vi "Set LabVIEW Server ID.vi"(7 "Server Alias":string, 10 "Error In":errorcluster, 11 "LabVIEW Server ID":string) -> (2 "Error Out":errorcluster)   [LabVIEW 2013, in "TS.lvlib"]
uses:
  TS.lvlib
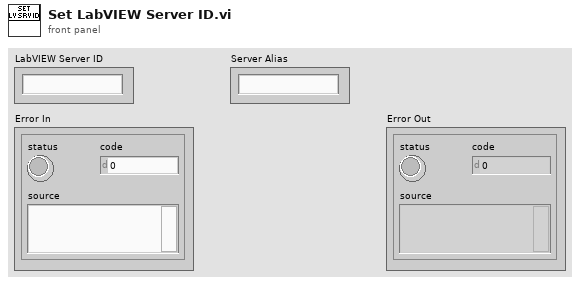
[diagram p1: front panel]
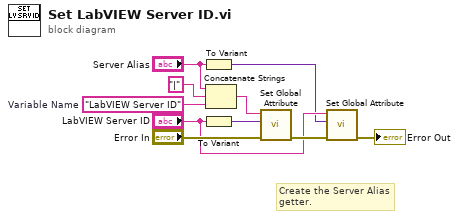
[diagram p0: block diagram]
diagram:
  w8 = "LabVIEW Server ID"  # Variable Name
  # "Create the Server Alias\ngetter."
  n1 = To Variant(anything="Server Alias") -> (Variant=w2:variant)
  n2 = To Variant(anything="LabVIEW Server ID") -> (Variant=w6:variant)
  n3 = Concatenate Strings("Server Alias", "|" ("string"), w8) -> (w7:string)
  n4 = call "Set Global Attribute.vi"("Error In"="Error In", "Value"=w6, "Name"=w7) -> ("Error Out"=w5:errorcluster)  [unwired: 7 in, 1 out]
  n5 = call "Set Global Attribute.vi"("Error In"=w5, "Value"=w2, "Name"="LabVIEW Server ID") -> ("Error Out"=→"Error Out":errorcluster)  [unwired: 7 in, 1 out]
